vi "Resitance.vi"(1 "I":dbl caption="I[A]", 2 "U":dbl caption="U[V]") -> (0 "R":dbl caption="R[Ohm]")   [LabVIEW 2020]
doc: "Liczy opór na podstawie prądu i napięcia."
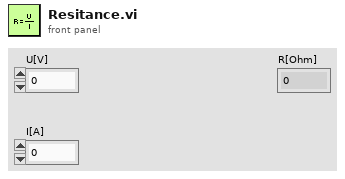
[diagram p1: front panel]
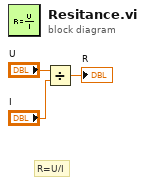
[diagram p0: block diagram]
diagram:
  # "R=U/I"
  n1 = Divide(x="U", y="I") -> (x/y=→"R":dbl)
